vi "AIT 664 - Extract Output VLs from System Explorer.vi"(0 "664 End System":T6, 5 "Item Ref in":T5 format="%.0x", 11 "error in (no error)":errorcluster) -> (4 "Output VLs out":T1[](array[typedef]), 15 "error out":errorcluster)   [LabVIEW 2013, in "AIT 664 Custom Device.lvlib"]
doc: "Extract the Output VLs from the system explorer and return the parameters defined by the user"
uses:
  AIT 664 Custom Device.lvlib
  Controls/664 - XML End System Description.ctl
  Controls/664 - XML Output VL.ctl
  Controls/664 - XML Tx Message Port.ctl
  Controls/664 - Sampling Type.ctl
  Controls/664 -Param.ctl
  Controls/664 - XML Input VL.ctl
  Controls/664 - XML Rx Message Port.ctl
  <vilib>/NI Veristand/Custom Device API/Custom Device Item Ref.ctl
  Controls and Global/Global.vi
  <vilib>/NI Veristand/Custom Device Tools/Custom Device Utility Library/NI VeriStand - Search for All Items by GUID.vi
  <vilib>/NI Veristand/Custom Device API/Get Item Property (U32).vi
  <vilib>/NI Veristand/Custom Device Tools/Custom Device Utility Library/Custom Device Utility Library.lvlib
  <vilib>/NI Veristand/Custom Device API/Custom Device API.lvlib
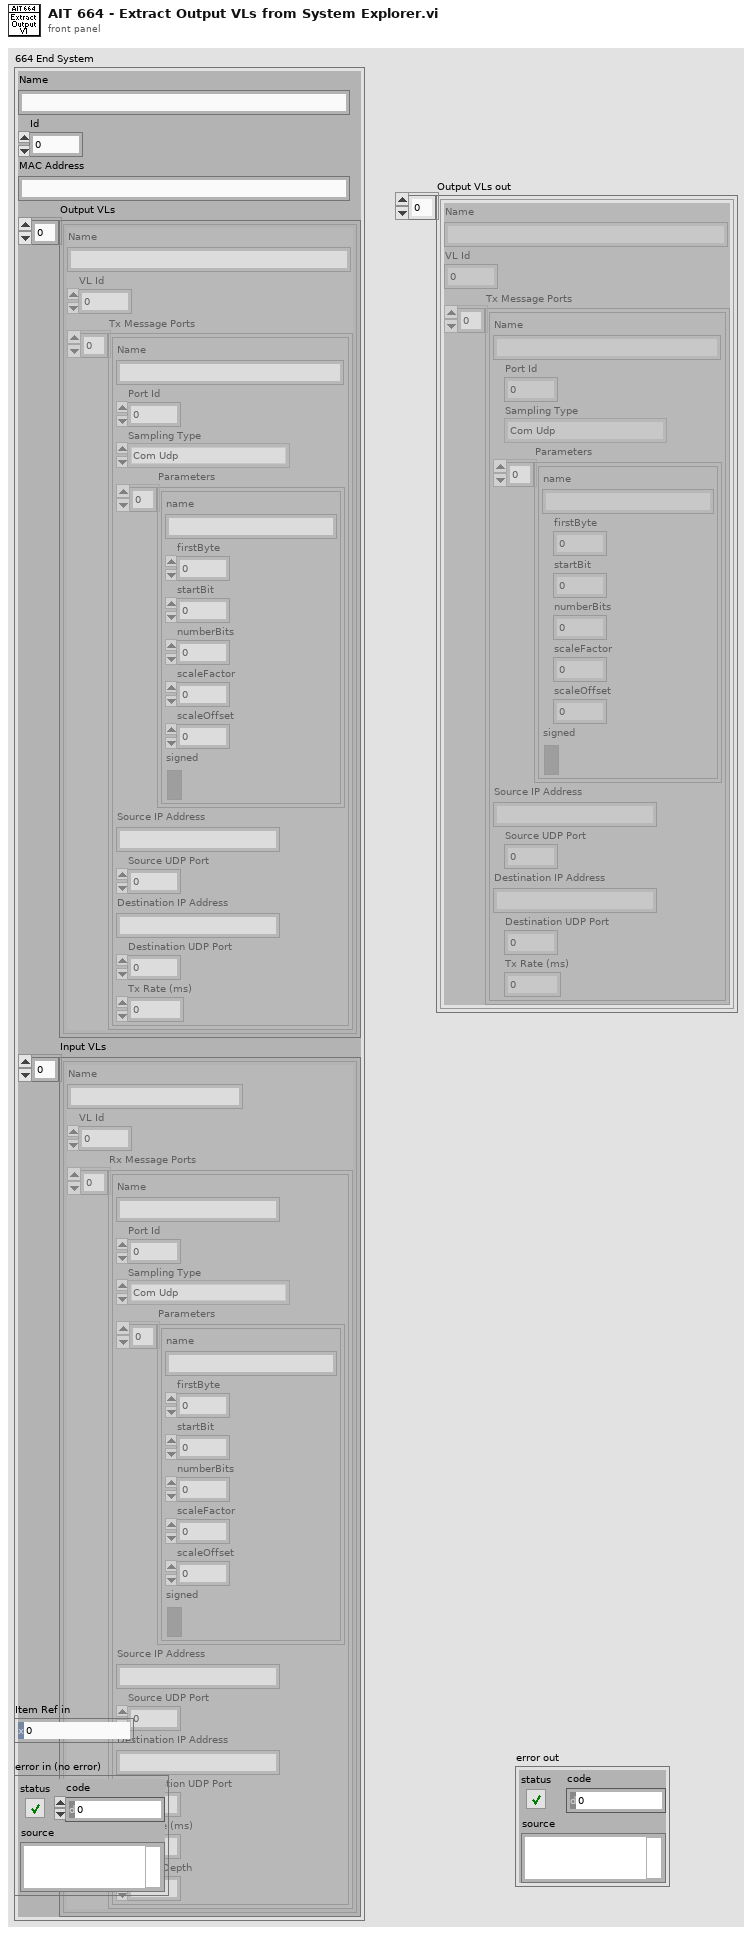
[diagram p1: front panel]
types:
  T1 = typedef "AIT 664 Custom Device.lvlib/664 - XML Output VL.ctl" = cluster{"Name":string, "VL Id":u32, "Tx Message Ports":T2[]}
  T2 = typedef "AIT 664 Custom Device.lvlib/664 - XML Tx Message Port.ctl" = cluster{"Name":string, "Port Id":u32, "Sampling Type":T3, "Parameters":T4[], "Source IP Address":string, "Source UDP Port":u32, "Destination IP Address":string, "Destination UDP Port":u32, "Tx Rate (ms)":u32}
  T3 = typedef "AIT 664 Custom Device.lvlib/664 - Sampling Type.ctl" = enum16{"Com Udp", "Com Udp Queuing", "Sap Udp", "Sap Ip", "Sap Mac", "Unknown"}
  T4 = typedef "AIT 664 Custom Device.lvlib/664 -Param.ctl" = cluster{"name":string, "firstByte":i32, "startBit":i32, "numberBits":i32, "scaleFactor":dbl, "scaleOffset":dbl, "signed":bool}
  T5 = typedef "Custom Device API.lvlib/Custom Device Item Ref.ctl" = u64
  T6 = typedef "AIT 664 Custom Device.lvlib/664 - XML End System Description.ctl" = cluster{"Name":string, "Id":u32, "MAC Address":string, "Output VLs":T1[], "Input VLs":T7[]}
  T7 = typedef "AIT 664 Custom Device.lvlib/664 - XML Input VL.ctl" = cluster{"Name":string, "VL Id":u32, "Rx Message Ports":T8[]}
  T8 = typedef "AIT 664 Custom Device.lvlib/664 - XML Rx Message Port.ctl" = cluster{"Name":string, "Port Id":u32, "Sampling Type":T3, "Parameters":T4[], "Source IP Address":string, "Source UDP Port":u32, "Destination IP Address":string, "Destination UDP Port":u32, "Rx Rate (ms)":u32, "Buffer Depth":u32}
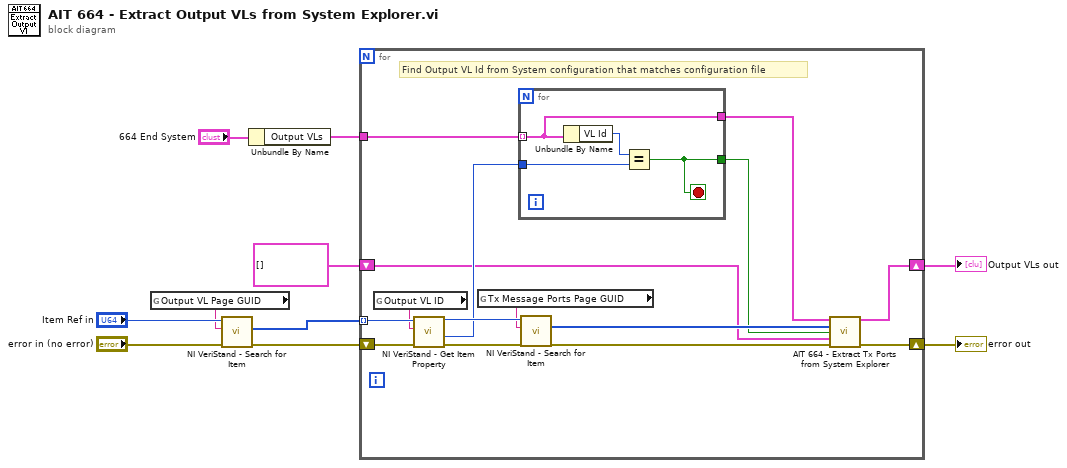
[diagram p0: block diagram]
diagram:
  n1 = global read "Global.vi" "Output VL Page GUID"() -> (w2:string)
  n2 = call-poly <vilib>:"NI VeriStand - Search for Item.vi"("error in"="error in (no error)", "Item GUID"=w2, "Section Ref in"="Item Ref in") -> ("error out"=w7:errorcluster, "Item Refs"=w3:T5[])  [unwired: 5 in, 2 out]
  n3 = Unbundle By Name("664 End System") -> ("Output VLs"=w4:T1[])
  n4 = for {
    tunnel: w3 -> [w25] mode=indexing
    tunnel: w4 -> [w19]
    shift-right: [w14] -> w5
    shift-left: T1[] [] -> [w15]
    shift-right: [w12] -> w1
    shift-left: w7 -> [w11]
    # "Find Output VL Id from System configuration that matches configuration file"
    n5 = global read "Global.vi" "Output VL ID"() -> (w24:string)
    n6 = call-poly <vilib>:"NI VeriStand - Get Item Property.vi"("error in (no error)"=w11, "Property Name"=w24, "Item Ref in"=w25) -> ("error out"=w23:errorcluster, "Value"=w18:u32, "Item Ref out"=w22:T5)  [unwired: 5 in, 1 out]
    n7 = global read "Global.vi" "Tx Message Ports Page GUID"() -> (w21:string)
    n8 = for {
      tunnel: w19 -> [w26] mode=indexing
      tunnel: w18 -> [w28]
      tunnel: [w27] -> w17
      tunnel: [w26] -> w16
      stop <- w27 stop-if-true
      n9 = Unbundle By Name(w26) -> ("VL Id"=w29:u32)
      n10 = Equal?(x=w29, y=w28) -> (x = y?=w27:bool)
    }
    n11 = call-poly <vilib>:"NI VeriStand - Search for Item.vi"("error in"=w23, "Item GUID"=w21, "Section Ref in"=w22) -> ("error out"=w13:errorcluster, "Item Refs"=w20:T5[])  [unwired: 5 in, 2 out]
    n12 = call "AIT 664 - Extract Tx Ports from System Explorer.vi"("Found Output VL"=w16, "Item Refs"=w20, "VL Id Found?"=w17, "Output VLs"=w15, "error in (no error)"=w13) -> ("Output VLs out"=w14:T1[], "error out"=w12:errorcluster)  [unwired: 9 in]
  }
  "Output VLs out" <- w5
  "error out" <- w1
